vi "EXCOM_33.vi"(0 "VISA resource name":refnum<visa-resource-name>, 1 "Bool Refnum":refnum<vi>, 11 "Error IN":errorcluster) -> (3 "Vtel":dbl format="%.1f", 4 "VISA resource name dup":refnum<visa-resource-name>, 14 "OK Done":bool=TRUE, 15 "error out":errorcluster)   [LabVIEW 2011]
panel:
  out "Q String":string="1\r108\r0\r"
  # "3 = COM4"
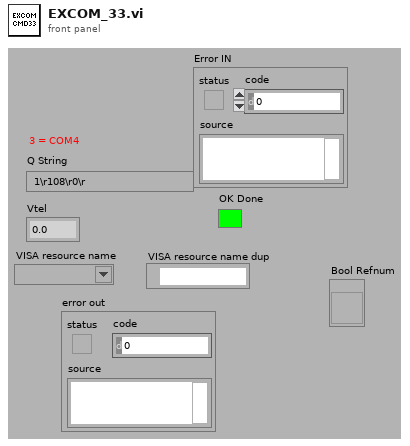
[diagram p1: front panel]
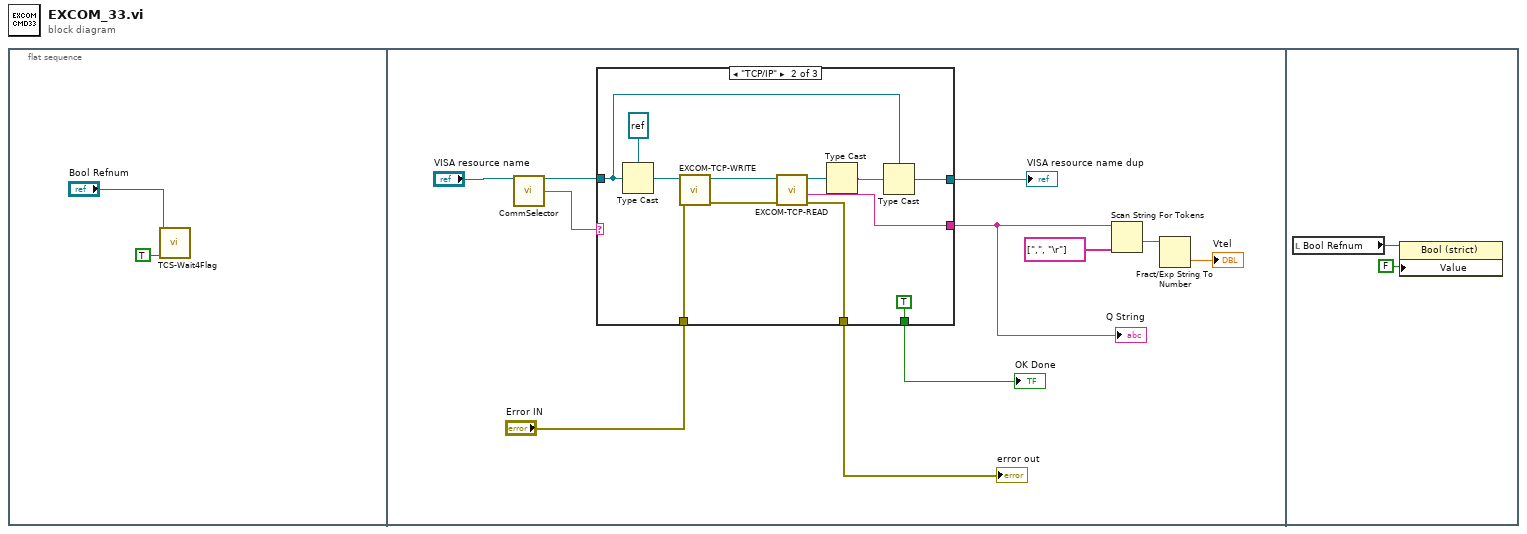
[diagram p0: block diagram]
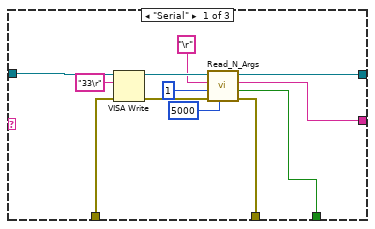
[diagram p2: hidden frame]
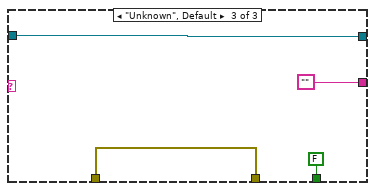
[diagram p3: hidden frame]
diagram:
  n1 = flat-sequence {
    frame #0 {
      n2 = call "TCS-Wait4Flag.vi"("Raise Flag ?"=TRUE, "Ctl Refnum IN"="Bool Refnum") -> ()  [unwired: 8 in, 2 out]
    }
    frame #1 {
      n3 = call "CommSelector.vi"("VISA resource name"="VISA resource name") -> ("VISA resource name"=w9:refnum<visa-resource-name>, "CommType"=w7:string)  [unwired: 13 in]
      n4 = case shown="\"TCP/IP\"" w7 {
        tunnel: [w14 TRUE ("OK Done") FALSE ("OK Done")] -> w13
        tunnel: w9 -> [w25 w31 w40]
        tunnel: [w15 w28 w39] -> w12
        tunnel: [w23 w32 w40] -> w11
        tunnel: "Error IN" -> [w21 w30 w39]
        tunnel: [w16 w26 ""] -> w3
        frame "Serial" {
          n5 = VISA Write(VISA resource name=w25, write buffer="33\r", error in (no error)=w21) -> (VISA resource name out=w24:refnum<visa-resource-name>, error out=w22:errorcluster)  [unwired: 1 out]
          n6 = call "Read_N_Args.vi"("Delay (ms)"=u32 5000, "Error IN"=w22, "Nb_Args"=1, "Arg_Char"="\r", "VRN IN"=w24) -> ("Error OUT"=w15:errorcluster, "All_Args?"=w14:bool, "Answer"=w16:string, "VRN OUT"=w23:refnum<visa-resource-name>)  [unwired: 3 in]
        }
        frame "TCP/IP" {
          n7 = Type Cast(type=refnum<k5> refnum ("connection ID out"), x=w31) -> (*(type *) &x=w37:refnum<k5>)
          n8 = call "EXCOM-TCP-WRITE.vi"("Error IN"=w30, "connection ID"=w37) -> ("Error OUT"=w29:errorcluster, "connection ID out"=w35:refnum<k5>)  [unwired: 5 in, 2 out]
          n9 = call "EXCOM-TCP-READ.vi"("Error In"=w29, "connection ID"=w35) -> ("Error Out"=w28:errorcluster, "Response"=w26:string, "CID Out"=w34:refnum<k5>)  [unwired: 5 in]
          n10 = Type Cast(x=w34) -> (*(type *) &x=w33:string)  [unwired: 1 in]
          n11 = Type Cast(type=w31, x=w33) -> (*(type *) &x=w32:refnum<visa-resource-name>)
        }
        frame "Unknown", Default {
        }
      }
      "OK Done" <- w13
      "error out" <- w12
      "VISA resource name dup" <- w11
      "Q String" <- w3
      n12 = Scan String For Tokens(6:string[] [",", "\r"] ("delimiters (\\s,\\t,\\r,\\n)"), 9:w3) -> (1:w6:string)  [unwired: 4 in, 3 out]
      n13 = Fract/Exp String To Number(string=w6) -> (number=→"Vtel":dbl)  [unwired: 3 in, 1 out]
    }
    frame #2 {
      n14 = local read "Bool Refnum"() -> (w43:refnum<vi>)
      n15 = property class="Bool (strict)"(reference=w43, "Value"=FALSE) -> ()  [unwired: 1 in, 2 out]
    }
  }
